vi "布尔复位型入队.vi"(0 "队列输入":refnum<queue>, 1 "数值":i32, 2 "控件引用":refnum<vi>, 3 "字符消息入队列":string) -> (5 "队列输出":refnum<queue>, 7 "控件引用 2":refnum<vi>, 8 "字符消息出队列":string)   [LabVIEW 2018]
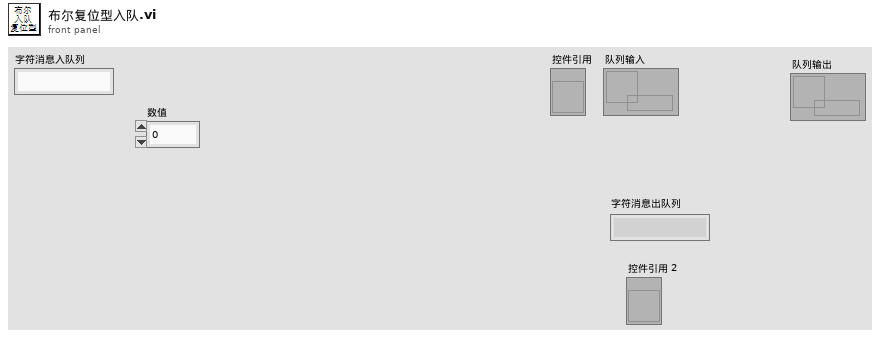
[diagram p1: front panel]
types:
  T1 = enum8{"Enabled", "Disabled", "Disabled and Grayed Out"}
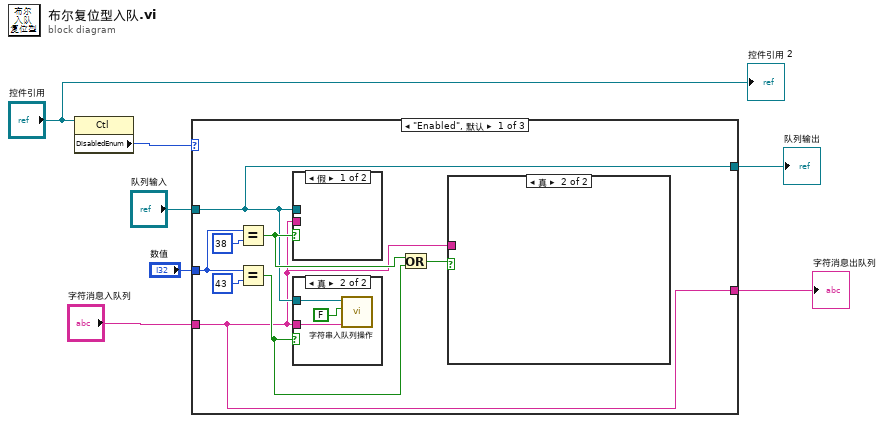
[diagram p0: block diagram]
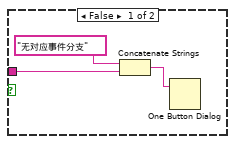
[diagram p2: hidden frame]
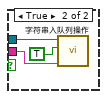
[diagram p4: hidden frame]
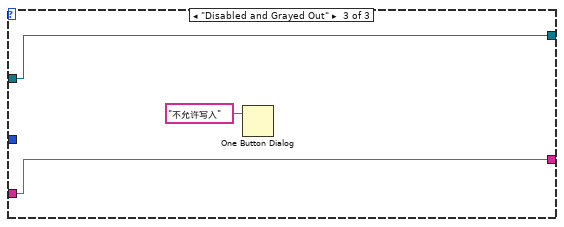
[diagram p6: hidden frame]
diagram:
  n1 = property class="Ctl"(reference="控件引用") -> ("DisabledEnum"=w7:T1)  [unwired: 1 in, 2 out]
  n2 = case shown="\"Enabled\", 默认" w7 {
    tunnel: "数值" -> [w13 _ _]
    tunnel: "队列输入" -> [w9 w26 w28]
    tunnel: "字符消息入队列" -> [w8 w25 w27]
    tunnel: [w9 w26 w28] -> w3
    tunnel: [w8 w25 w27] -> w2
    frame "Enabled", Default {
      n3 = Equal?(x=w13, y=38) -> (x = y?=w12:bool)
      n4 = Equal?(x=w13, y=43) -> (x = y?=w11:bool)
      n5 = case shown="假" w12 {
        tunnel: w9 -> [_ w24]
        tunnel: w8 -> [_ w22]
        frame False {
        }
        frame True {
          n6 = call "字符串入队列操作.vi"("字符消息入队列"=w22, "布尔"=TRUE, "界面切换队列"=w24) -> ()  [unwired: 8 in, 1 out]
        }
      }
      n7 = case shown="真" w11 {
        tunnel: w9 -> [_ w21]
        tunnel: w8 -> [_ w19]
        frame False {
        }
        frame True {
          n8 = call "字符串入队列操作.vi"("字符消息入队列"=w19, "布尔"=FALSE, "界面切换队列"=w21) -> ()  [unwired: 8 in, 1 out]
        }
      }
      n9 = Or(x=w12, y=w11) -> (x .or. y?=w10:bool)
      n10 = case shown="真" w10 {
        tunnel: w8 -> [w18 _]
        frame False {
          n11 = Concatenate Strings("无对应事件分支" ("字符串"), w18) -> (w16:string)
          n12 = One Button Dialog(message=w16) -> ()  [unwired: 1 in, 1 out]
        }
        frame True {
        }
      }
    }
    frame "Disabled" {
    }
    frame "Disabled and Grayed Out" {
      n13 = One Button Dialog(message="不允许写入" ("消息")) -> ()  [unwired: 1 in, 1 out]
    }
  }
  "队列输出" <- w3
  "字符消息出队列" <- w2
  "控件引用 2" <- "控件引用"
